vi "Update Control Based on Key Down.vi"(6 "PlatMods":T5, 9 "VKey":T6, 10 "Refnums for Resizing and Alignment in":T1, 11 "display state in":T2={"Graph Visible Items"={"Plot Legend"=FALSE, "Scale Legend"=FALSE, "Graph Palette"=FALSE, "Cursor Legend"=FALSE, "X Scrollbar"=FALSE}, "View Table"=FALSE, "Table Visible Items"={"Vertical Scrollbar"=FALSE, "Horizontal Scrollbar"=FALSE, "Row Headers"=FALSE, "Column Headers"=FALSE, "Vertical Lines"=FALSE, "Horizontal Lines"=FALSE}, "Header Font"={"Font Name"="", "Size"=0, "Bold"=FALSE, "Italic"=FALSE, "Underline"=FALSE, "Strikeout"=FALSE, "Color"=0}, "Cell Font"={"Font Name"="", "Size"=0, "Bold"=FALSE, "Italic"=FALSE, "Underline"=FALSE, "Strikeout"=FALSE, "Color"=0}, "Description and Tip..."={"Description"="", "Tip"=""}, "Moveable Splitter Position"=0, "Measurement Cursor Configuration"={"XY"={"enable XY"=FALSE, "Position (X)"=[], "Type"=enum."Absolute", "Y reference"=0.0, "color"=0}, "band"={"enable band"=FALSE, "B1"=0.0, "B2"=0.0, "Fixed bandwidth (B2-B1)"=0.0, "B1 color"=0, "B2 color"=0}, "harmonic"={"enable harmonics"=FALSE, "X reference (1X)"=0.0, "Maximum"=0, "Subset"=enum."All", "1X color"=0, "MX color"=0}, "sideband"={"enable sideband"=FALSE, "X center (C)"=0.0, "Sidebands"=0, "X spacing (s)"=0.0, "Center color"=0, "Sideband color"=0}}, "Cursors"={"List"=[], "Tags"=[]}, "X Increment"=0.0, "X Scale"={"Label Visible"=FALSE, "Label Text"="", "Mapping Mode"=0, "Format String"=""}, "Y Scale"={"Label Visible"=FALSE, "Label Text"="", "Mapping Mode"=0, "Format String"=""}, "Colors"={"background"=16777215, "major grid"=8355711, "minor grid"=12632256, "font"=0}, "desired spectrum view"={"scaling"={"linear/dB"=enum."no change", "dB reference"=0.0, "power/magnitude"=enum."no change", "view"=enum."no change"}, "spectral density"=enum."no change"}, "Plot Color Wheel"=[3381759, 32768, 982784, 4375295, 13827953, 13457919, 16757522, 4343295, 16728758, 12095254], "Plots"=[], "registered user events"=variant, "Lock 1X to Peak"=FALSE} caption="State" {"Y Scale"."Mapping Mode" items=["Linear", "Logarithmic", "dB"]; "X Scale"."Mapping Mode" items=["Linear", "Logarithmic"]}) -> (0 "Position.X":dbl, 1 "selected cursor":string, 2 "Refnums for Resizing and Alignment out":T1, 3 "display state out":T2={"Graph Visible Items"={"Plot Legend"=FALSE, "Scale Legend"=FALSE, "Graph Palette"=FALSE, "Cursor Legend"=FALSE, "X Scrollbar"=FALSE}, "View Table"=FALSE, "Table Visible Items"={"Vertical Scrollbar"=FALSE, "Horizontal Scrollbar"=FALSE, "Row Headers"=FALSE, "Column Headers"=FALSE, "Vertical Lines"=FALSE, "Horizontal Lines"=FALSE}, "Header Font"={"Font Name"="", "Size"=0, "Bold"=FALSE, "Italic"=FALSE, "Underline"=FALSE, "Strikeout"=FALSE, "Color"=0}, "Cell Font"={"Font Name"="", "Size"=0, "Bold"=FALSE, "Italic"=FALSE, "Underline"=FALSE, "Strikeout"=FALSE, "Color"=0}, "Description and Tip..."={"Description"="", "Tip"=""}, "Moveable Splitter Position"=0, "Measurement Cursor Configuration"={"XY"={"enable XY"=FALSE, "Position (X)"=[], "Type"=enum."Absolute", "Y reference"=0.0, "color"=0}, "band"={"enable band"=FALSE, "B1"=0.0, "B2"=0.0, "Fixed bandwidth (B2-B1)"=0.0, "B1 color"=0, "B2 color"=0}, "harmonic"={"enable harmonics"=FALSE, "X reference (1X)"=0.0, "Maximum"=0, "Subset"=enum."All", "1X color"=0, "MX color"=0}, "sideband"={"enable sideband"=FALSE, "X center (C)"=0.0, "Sidebands"=0, "X spacing (s)"=0.0, "Center color"=0, "Sideband color"=0}}, "Cursors"={"List"=[], "Tags"=[]}, "X Increment"=0.0, "X Scale"={"Label Visible"=FALSE, "Label Text"="", "Mapping Mode"=0, "Format String"=""}, "Y Scale"={"Label Visible"=FALSE, "Label Text"="", "Mapping Mode"=0, "Format String"=""}, "Colors"={"background"=16777215, "major grid"=8355711, "minor grid"=12632256, "font"=0}, "desired spectrum view"={"scaling"={"linear/dB"=enum."no change", "dB reference"=0.0, "power/magnitude"=enum."no change", "view"=enum."no change"}, "spectral density"=enum."no change"}, "Plot Color Wheel"=[3381759, 32768, 982784, 4375295, 13827953, 13457919, 16757522, 4343295, 16728758, 12095254], "Plots"=[], "registered user events"=variant, "Lock 1X to Peak"=FALSE} caption="State" {"Y Scale"."Mapping Mode" items=["Linear", "Logarithmic", "dB"]; "X Scale"."Mapping Mode" items=["Linear", "Logarithmic"]}, 4 "discard?":bool)   [LabVIEW 2017, in "Octave with Cursors.xctl"]
doc: "On left/right arrow, move the selected cursor and update the table value.\nOn up/down arrow, increment the cursor selection."
uses:
  <vilib>/addons/_XControls/Octave with Cursors/Octave with Cursors.xctl
  <vilib>/addons/_XControls/Octave with Cursors/Controls/Refnums Typedef.ctl
  <vilib>/addons/Sound and Vibration/svt_Controls/subVIs/Multiplot Octave Graph.ctl
  <vilib>/event_ctls.llb/eventvkey.ctl
  <vilib>/addons/_XControls/Octave with Cursors/Controls/State.ctl
  <vilib>/Utility/miscctls.llb/LVFontTypeDef.ctl
  <vilib>/addons/_XControls/Octave with Cursors/Controls/Measurement Cursor Configuration.ctl
  <vilib>/Utility/miscctls.llb/LVRowAndColumnTypeDef.ctl
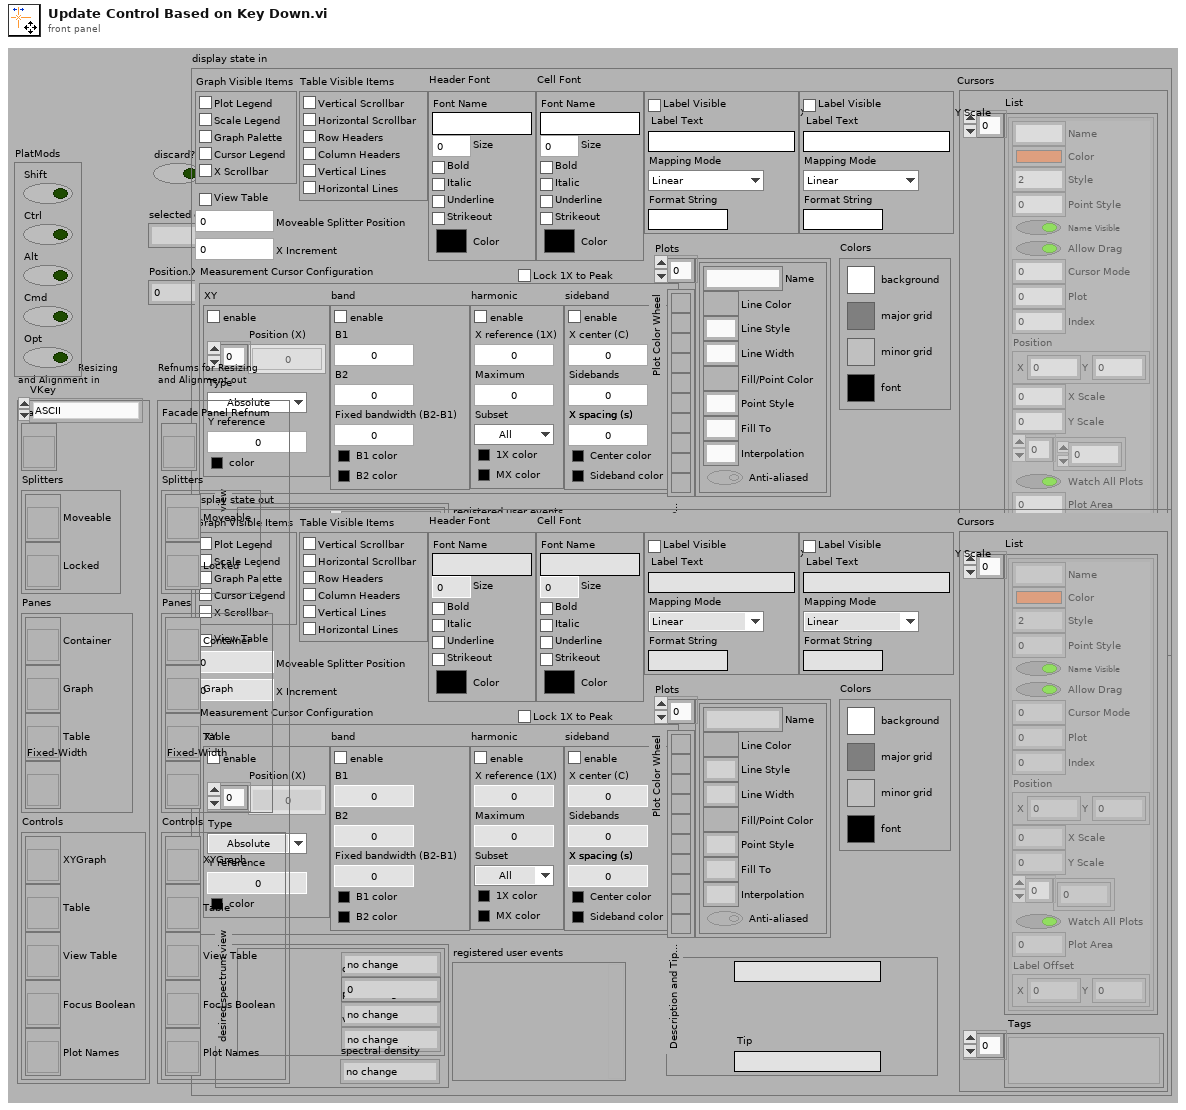
[diagram p1: front panel]
types:
  T1 = typedef "Octave with Cursors.xctl/Refnums Typedef.ctl" = cluster{"Facade Panel Refnum":refnum<vi>, "Splitters":cluster{"Moveable":refnum<vi>, "Locked":refnum<vi>}, "Panes":cluster{"Container":refnum<vi>, "Graph":refnum<vi>, "Table":refnum<vi>, "Fixed-Width":refnum<vi>}, "Controls":cluster{"XYGraph":refnum<vi>, "Table":refnum<vi>, "View Table":refnum<vi>, "Focus Boolean":refnum<vi>, "Plot Names":refnum<vi>}}
  T2 = typedef "Octave with Cursors.xctl/State.ctl" = cluster{"Graph Visible Items":cluster{"Plot Legend":bool, "Scale Legend":bool, "Graph Palette":bool, "Cursor Legend":bool, "X Scrollbar":bool}, "View Table":bool, "Table Visible Items":cluster{"Vertical Scrollbar":bool, "Horizontal Scrollbar":bool, "Row Headers":bool, "Column Headers":bool, "Vertical Lines":bool, "Horizontal Lines":bool}, "Header Font":T3, "Cell Font":T3, "Description and Tip...":cluster{"Description":string, "Tip":string}, "Moveable Splitter Position":i32, "Measurement Cursor Configuration":T4, "Cursors":cluster{"List":cluster{"Name":string, "Color":u32, "Style":i32, "Point Style":u8, "Name Visible":bool, "Allow Drag":bool, "Cursor Mode":u32, "Plot":i32, "Index":i32, "Position":cluster{"X":dbl, "Y":dbl}, "X Scale":u32, "Y Scale":u32, "Watch Plots":i32[], "Watch All Plots":bool, "Plot Area":i32, "Label Offset":cluster{"X":dbl, "Y":dbl}}[], "Tags":variant[]}, "X Increment":dbl, "X Scale":cluster{"Label Visible":bool, "Label Text":string, "Mapping Mode":u8, "Format String":string}, "Y Scale":cluster{"Label Visible":bool, "Label Text":string, "Mapping Mode":u8, "Format String":string}, "Colors":cluster{"background":u32, "major grid":u32, "minor grid":u32, "font":u32}, "desired spectrum view":cluster{"scaling":cluster{"linear/dB":enum16{"no change", "linear", "dB"}, "dB reference":dbl, "power/magnitude":enum16{"no change", "power", "magnitude"}, "view":enum16{"no change", "rms", "peak", "peak-peak"}}, "spectral density":enum16{"no change", "spectrum", "spectral density"}}, "Plot Color Wheel":u32[], "Plots":cluster{"Name":string, "Line Color":u32, "Line Style":u8, "Line Width":u8, "Fill/Point Color":u32, "Point Style":u8, "Fill To":i16, "Interpolation":u8, "Anti-aliased":bool}[], "registered user events":variant, "Lock 1X to Peak":bool}
  T3 = typedef "LVFontTypeDef.ctl" = cluster{"Font Name":string, "Size":u16, "Bold":bool, "Italic":bool, "Underline":bool, "Strikeout":bool, "Color":u32}
  T4 = typedef "Octave with Cursors.xctl/Measurement Cursor Configuration.ctl" = cluster{"XY":cluster{"enable XY":bool, "Position (X)":dbl[], "Type":enum16{"Absolute", "Relative"}, "Y reference":dbl, "color":u32}, "band":cluster{"enable band":bool, "B1":dbl, "B2":dbl, "Fixed bandwidth (B2-B1)":dbl, "B1 color":u32, "B2 color":u32}, "harmonic":cluster{"enable harmonics":bool, "X reference (1X)":dbl, "Maximum":i32, "Subset":enum16{"All", "Even", "Odd"}, "1X color":u32, "MX color":u32}, "sideband":cluster{"enable sideband":bool, "X center (C)":dbl, "Sidebands":i32, "X spacing (s)":dbl, "Center color":u32, "Sideband color":u32}}
  T5 = cluster{"Shift":bool, "Ctrl":bool, "Alt":bool, "Cmd":bool, "Opt":bool}
  T6 = typedef "eventvkey.ctl" = enum16{"ASCII", "Enter", "Return", "Shift", "Ctrl", "Alt", "Cmd", "Opt", "Caps", "NumLock", "Clear", "Break", "Up", "Down", "Left", "Right", "Insert", "Delete", "Home", "End", "PageUp", "PageDown", "Escape", "Help", "Pause", "ScrollLock", "F1", "F2", "F3", "F4", "F5", "F6", "F7", "F8", "F9", "F10", "F11", "F12", "F13", "F14", "F15", "F16", "F17", "F18", "F19", "F20", "F21", "F22", "F23", "F24", "Play", "VolumeUp", "VolumeDown", "Mute", "Two Byte Char"}
  T7 = typedef "LVRowAndColumnTypeDef.ctl" = cluster{"Row":i32, "Column":i32}
  T8 = cluster{"Name":string, "Color":u32, "Style":i32, "Point Style":u8, "Name Visible":bool, "Allow Drag":bool, "Cursor Mode":u32, "Plot":i32, "Index":i32, "Position":cluster{"X":dbl, "Y":dbl}, "X Scale":u32, "Y Scale":u32, "Watch Plots":i32[], "Watch All Plots":bool, "Plot Area":i32, "Label Offset":cluster{"X":dbl, "Y":dbl}}[]
  T9 = cluster{"Name":string, "Color":u32, "Style":i32, "Point Style":u8, "Name Visible":bool, "Allow Drag":bool, "Cursor Mode":u32, "Plot":i32, "Index":i32, "Position":cluster{"X":dbl, "Y":dbl}, "X Scale":u32, "Y Scale":u32, "Watch Plots":i32[], "Watch All Plots":bool, "Plot Area":i32, "Label Offset":cluster{"X":dbl, "Y":dbl}}
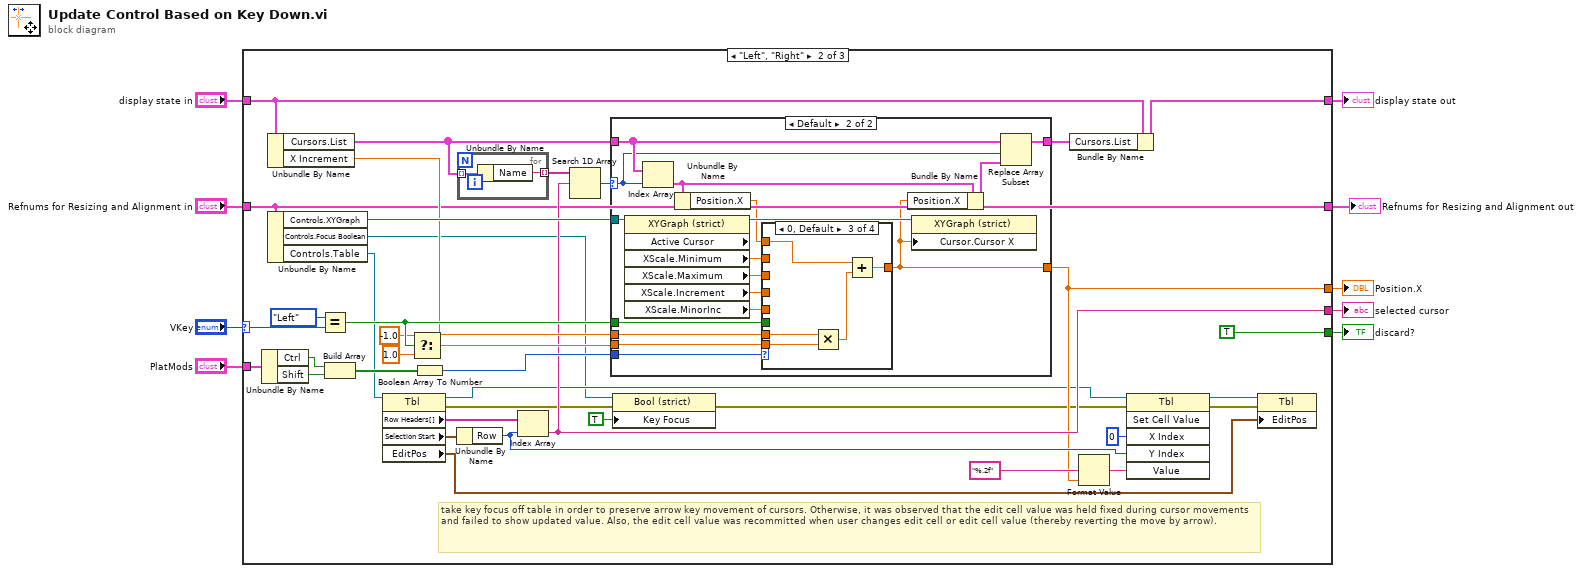
[diagram p0: block diagram]
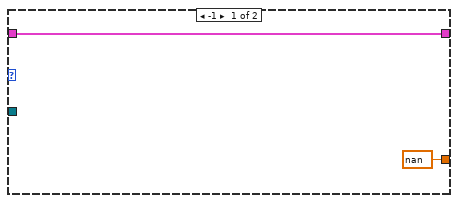
[diagram p3: hidden frame]
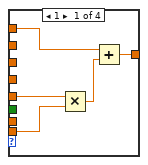
[diagram p4: hidden frame]
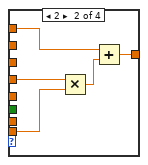
[diagram p5: hidden frame]
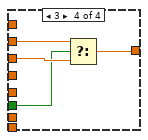
[diagram p6: hidden frame]
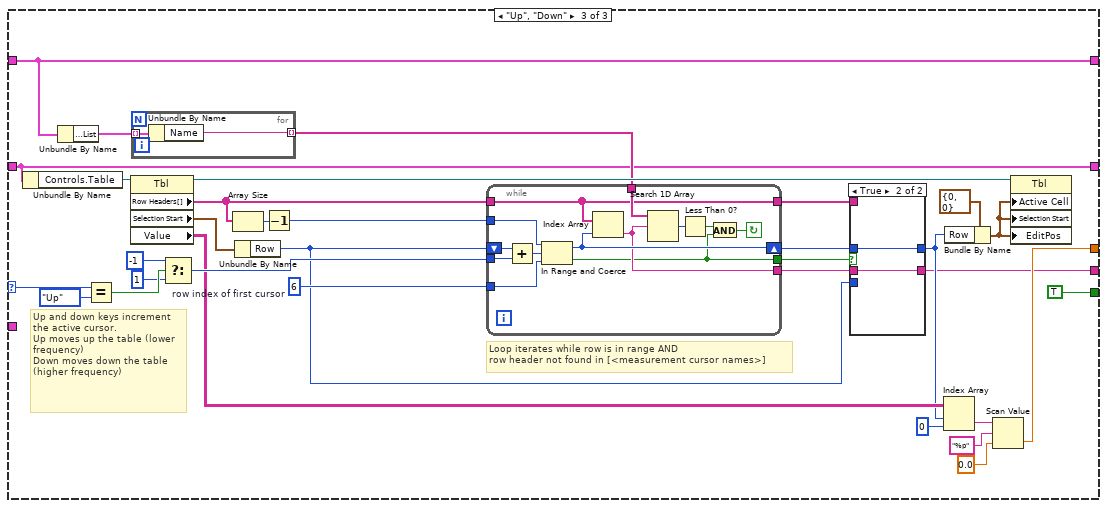
[diagram p7: hidden frame]
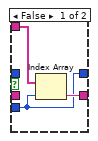
[diagram p8: hidden frame]
diagram:
  n1 = case shown="\"Left\", \"Right\"" "VKey" {
    selector: "VKey" -> [_ w47 w121]
    tunnel: [_ TRUE ("Key Focus") TRUE] -> w9
    tunnel: "PlatMods" -> [_ w41 _]
    tunnel: "Refnums for Resizing and Alignment in" -> [w10 w17 w90]
    tunnel: [_ w23 w109] -> w5
    tunnel: [_ w25 w94] -> w4
    tunnel: [w11 w18 w100] -> w3
    tunnel: "display state in" -> [w11 w19 w100]
    tunnel: [w10 w17 w90] -> w1
    frame Default {
    }
    frame "Left", "Right" {
      # "take key focus off table in order to preserve arrow key movement of cursors. Otherwise, it was observed that the edit cell value was held fixed during cursor movements and failed to show updated value. Also, the edit cell value was recommitted when user changes edit cell or edit cell value (thereby reverting the move by arrow)."
      n2 = Unbundle By Name(w41) -> ("Ctrl"=w40:bool, "Shift"=w39:bool)
      n3 = Unbundle By Name(w19) -> ("Cursors.List"=w21:T8, "X Increment"=w26:dbl)
      n4 = Unbundle By Name(w17) -> ("Controls.XYGraph"=w38:refnum<vi>, "Controls.Focus Boolean"=w14:refnum<vi>, "Controls.Table"=w37:refnum<vi>)
      n5 = Equal?(x=eventvkey."Left" ("VKey"), y=w47) -> (x = y?=w46:bool)
      n6 = Build Array(w40, w39) -> (w49:bool[])
      n7 = property class="Tbl"(reference=w37) -> (reference out=w15:refnum<vi>, error out=w16:errorcluster, "Row Headers[]"=w35:string[], "Selection Start"=w36:T7, "EditPos"=w28:T7)  [unwired: 1 in]
      n8 = Select(t=-1.0, s=w46, f=1.0) -> (s? t:f=w43:dbl)
      n9 = Boolean Array To Number(Boolean array=w49) -> (number=w48:u32)
      n10 = Unbundle By Name(w36) -> ("Row"=w31:i32)
      n11 = for {
        tunnel: w21 -> [w89] mode=indexing
        tunnel: [w88] -> w27 mode=indexing
        n12 = Unbundle By Name(w89) -> ("Name"=w88:string)
      }
      n13 = Index Array(array=w35, index=w31) -> (element=w25:string)
      n14 = Search 1D Array(1D array=w27, element=w25) -> (index of element=w22:i32)  [unwired: 1 in]
      n15 = case shown="Default" w22 {
        selector: w22 -> [_ w55]
        tunnel: w48 -> [_ w67]
        tunnel: w46 -> [_ w62]
        tunnel: w43 -> [_ w61]
        tunnel: w38 -> [_ w60]
        tunnel: w26 -> [_ w59]
        tunnel: [nan ("XScale.Maximum") w53] -> w23
        tunnel: w21 -> [w50 w58]
        tunnel: [w50 w57] -> w20
        frame -1 {
        }
        frame Default {
          n16 = property class="XYGraph (strict)" props=["Active Cursor", "XScale", "Minimum", "XScale", "Maximum", "XScale", "Increment", "XScale", "MinorInc"](reference=w60) -> (reference out=w68:refnum<vi>, "XScale.Minimum"=w66:dbl, "XScale.Maximum"=w65:dbl, "XScale.Increment"=w64:dbl, "XScale.MinorInc"=w63:dbl)  [unwired: 1 in, 2 out]
          n17 = Index Array(array=w58, index=w55) -> (element=w56:T9)
          n18 = Unbundle By Name(w56) -> ("Position.X"=w54:dbl)
          n19 = case shown="0, Default" w67 {
            tunnel: w62 -> [_ _ _ w85]
            tunnel: w66 -> [_ _ _ w87]
            tunnel: w65 -> [_ _ _ w86]
            tunnel: [w71 w74 w80 w84] -> w53
            tunnel: w64 -> [_ w77 _ _]
            tunnel: w63 -> [w73 _ _ _]
            tunnel: w54 -> [w70 w75 w81 _]
            tunnel: w61 -> [w72 w76 w82 _]
            tunnel: w59 -> [_ _ w79 _]
            frame 1 {
              n20 = Multiply(x=w73, y=w72) -> (x*y=w69:dbl)
              n21 = Add(x=w70, y=w69) -> (x+y=w71:dbl)
            }
            frame 2 {
              n22 = Multiply(x=w77, y=w76) -> (x*y=w78:dbl)
              n23 = Add(x=w75, y=w78) -> (x+y=w74:dbl)
            }
            frame 0, Default {
              n24 = Multiply(x=w79, y=w82) -> (x*y=w83:dbl)
              n25 = Add(x=w81, y=w83) -> (x+y=w80:dbl)
            }
            frame 3 {
              n26 = Select(t=w87, s=w85, f=w86) -> (s? t:f=w84:dbl)
            }
          }
          n27 = Bundle By Name(cluster=w56, "Position.X"=w53) -> (w52:T9)
          n28 = property class="XYGraph (strict)"(reference=w68, "Cursor.Cursor X"=w53) -> ()  [unwired: 1 in, 2 out]
          n29 = Replace Array Subset(array=w58, new element=w52, index=w55) -> (w57:T8)
        }
      }
      n30 = property class="Bool (strict)"(reference=w14, error in=w16, "Key Focus"=TRUE) -> (error out=w13:errorcluster)  [unwired: 1 out]
      n31 = Bundle By Name(cluster=w19, "Cursors.List"=w20) -> (w18:T2)
      n32 = Format Value(format string="%.2f", value (0)=w23) -> (output string=w33:string)  [unwired: 1 in]
      n33 = invoke class="Tbl" method="Set Cell Value"(reference=w15, error in=w13, "X Index"=u32 0, "Y Index"=w31, "Value"=w33) -> (reference out=w30:refnum<vi>, error out=w29:errorcluster)  [unwired: 1 in, 4 out]
      n34 = property class="Tbl"(reference=w30, error in=w29, "EditPos"=w28) -> ()  [unwired: 2 out]
    }
    frame "Up", "Down" {
      w101 = 6  # row index of first cursor
      # "Loop iterates while row is in range AND \nrow header not found in [<measurement cursor names>]"
      # "Up and down keys increment the active cursor.\nUp moves up the table (lower frequency)\nDown moves down the table (higher frequency)"
      n35 = Unbundle By Name(w90) -> ("Controls.Table"=w116:refnum<vi>)
      n36 = Unbundle By Name(w100) -> ("Cursors.List"=w99:T8)
      n37 = Equal?(x=w121, y=eventvkey."Up" ("VKey")) -> (x = y?=w119:bool)
      n38 = property class="Tbl"(reference=w116) -> (reference out=w120:refnum<vi>, "Row Headers[]"=w102:string[], "Selection Start"=w103:T7, "Value"=w108:string[][])  [unwired: 1 in, 1 out]
      n39 = for {
        tunnel: w99 -> [w142] mode=indexing
        tunnel: [w141] -> w98 mode=indexing
        n40 = Unbundle By Name(w142) -> ("Name"=w141:string)
      }
      n41 = Select(t=-1 ("lower limit"), s=w119, f=1 ("lower limit")) -> (s? t:f=w113:i32)
      n42 = Array Size(array=w102) -> (size(s)=w118:i32)
      n43 = Unbundle By Name(w103) -> ("Row"=w92:i32)
      n44 = Decrement(x=w118) -> (x-1=w106:i32)
      n45 = while {
        tunnel: w106 -> [w140]
        tunnel: w113 -> [w139]
        tunnel: w102 -> [w128]
        tunnel: [w133] -> w93
        shift-right: [w136] -> w95
        shift-left: w92 -> [w137]
        tunnel: w101 -> [w130]
        tunnel: w98 -> [w135]
        tunnel: [w129] -> w97
        tunnel: [w128] -> w91
        stop <- w134 continue-if-true
        n46 = Add(x=w137, y=w139) -> (x+y=w138:i32)
        n47 = In Range and Coerce(upper limit=w140, x=w138, lower limit=w130) -> (coerced(x)=w136:i32, In Range?=w129:bool)
        n48 = Index Array(array=w128, index=w136) -> (element=w133:string)
        n49 = Search 1D Array(1D array=w135, element=w133) -> (index of element=w132:i32)  [unwired: 1 in]
        n50 = Less Than 0?(x=w132) -> (x < 0?=w131:bool)
        n51 = And(x=w131, y=w129) -> (x .and. y?=w134:bool)
      }
      n52 = case shown="True" w97 {
        tunnel: [w123 w127] -> w96
        tunnel: w95 -> [_ w127]
        tunnel: [w124 w126] -> w94
        tunnel: w93 -> [_ w126]
        tunnel: w92 -> [w123 _]
        tunnel: w91 -> [w125 _]
        frame False {
          n53 = Index Array(array=w125, index=w123) -> (element=w124:string)
        }
        frame True {
        }
      }
      n54 = Index Array(array=w108, index (row)=w96, index (col)=0 ("disabled index (col)")) -> (element=w112:string)
      n55 = Bundle By Name(cluster=T7 {"Row"=0, "Column"=0} ("Active Cell:Active Cell"), "Row"=w96) -> (w104:T7)
      n56 = Scan Value(string=w112, format string="%p", default (0 dbl)=0.0) -> (value=w109:dbl)  [unwired: 1 out]
      n57 = property class="Tbl"(reference=w120, "Active Cell"=w104, "Selection Start"=w104, "EditPos"=w104) -> ()  [unwired: 1 in, 2 out]
    }
  }
  "discard?" <- w9
  "Position.X" <- w5
  "selected cursor" <- w4
  "display state out" <- w3
  "Refnums for Resizing and Alignment out" <- w1
